vi "Encoder Tick Distance.vi"(1 "Wheel Diameter":dbl, 2 "Encoder Lines":u16) -> (0 "Distance per Tick":dbl)   [LabVIEW 2015]
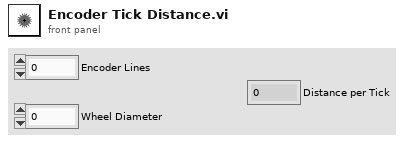
[diagram p1: front panel]
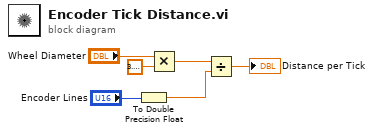
[diagram p0: block diagram]
diagram:
  n1 = To Double Precision Float(number="Encoder Lines") -> (double precision float=w2:dbl)
  n2 = Multiply(x="Wheel Diameter", y=3.141592653589793) -> (x*y=w4:dbl)
  n3 = Divide(x=w4, y=w2) -> (x/y=→"Distance per Tick":dbl)
